vi "SRV_PM_Segregate Data into Packets.vi"(0 "Array of Packets":T1[](array[typedef]) {"Packet Data" format="%.0x"}, 7 "Stuffed Data":u8[](array[numeric]) format="%.0x") -> (4 "Array of Packets out":T1[](array[typedef]) {"Packet Data" format="%.0x"})   [LabVIEW 2009]
uses:
  SRV_PM_Packet.ctl
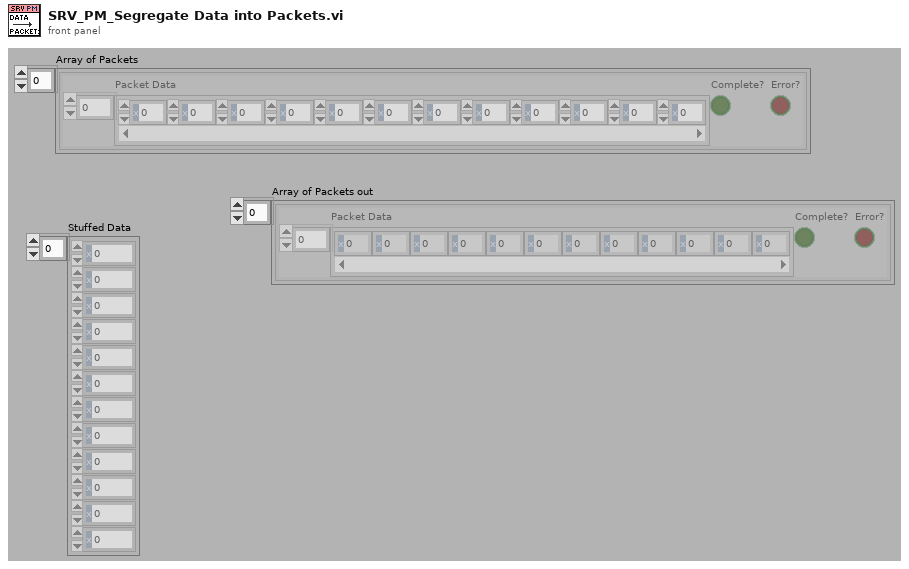
[diagram p1: front panel]
types:
  T1 = typedef "SRV_PM_Packet.ctl" = cluster{"Packet Data":u8[], "Complete?":bool, "Error?":bool}
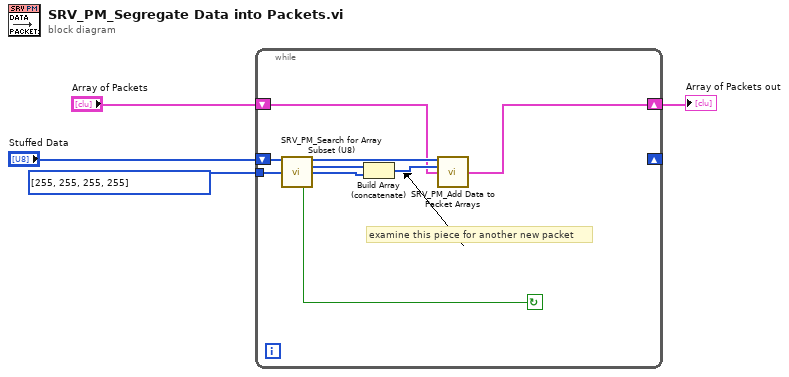
[diagram p0: block diagram]
diagram:
  n1 = while {
    tunnel: u8[] [255, 255, 255, 255] ("Search") -> [w12]
    shift-right: _ -> [_]
    shift-left: "Stuffed Data" -> [w13]
    shift-right: [w5] -> w1
    shift-left: "Array of Packets" -> [w6]
    stop <- w11 continue-if-true
    # "examine this piece for another new packet"
    n2 = call "SRV_PM_Search for Array Subset (U8).vi"("1D Array"=w13, "Search"=w12) -> ("Before Match"=w10:u8[], "Match"=w9:u8[], "After Match"=w8:u8[], "Found?"=w11:bool)  [unwired: 8 in, 2 out]
    n3 = Build Array (concatenate)(w9, w8) -> (w7:u8[])
    n4 = call "SRV_PM_Add Data to Packet Arrays.vi"("Previous Packet Data"=w10, "New Packet Data"=w7, "Array of Packets"=w6) -> ("Array of Packets out"=w5:T1[])  [unwired: 12 in]
  }
  "Array of Packets out" <- w1
